vi "Pre Launch Init.vi"(11 "Keepalive Heartbeat in":refnum<class "Keepalive Heartbeat.lvclass">) -> (0 "error out":errorcluster, 3 "Keepalive Heartbeat out":refnum<class "Keepalive Heartbeat.lvclass">)   [LabVIEW 2021, in "WebSocket Actors.lvlib" / "Keepalive Heartbeat.lvclass"]
doc: "(<B>Filename</B>: Actor Framework.lvlib:Actor.lvclass:Pre Launch Init.vi)\n\nDefines behavior that occurs after the Launch Nested Actor method is invoked but before the actor's Actor Core method begins running.\n\nBy default, this method does nothing. A descendant class may override it to define behavior."
uses:
  Keepalive Heartbeat.lvclass
  Keepalive Heartbeat.lvclass/Keepalive Heartbeat.ctl
  <vilib>/ActorFramework/Actor/Actor.lvclass
  <userlib>/_OpenG.lib/error/error.llb/openg_error.lvlib
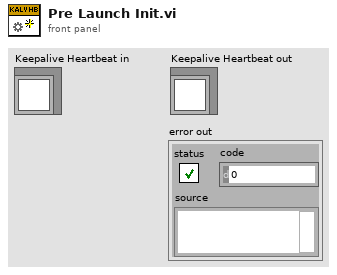
[diagram p1: front panel]
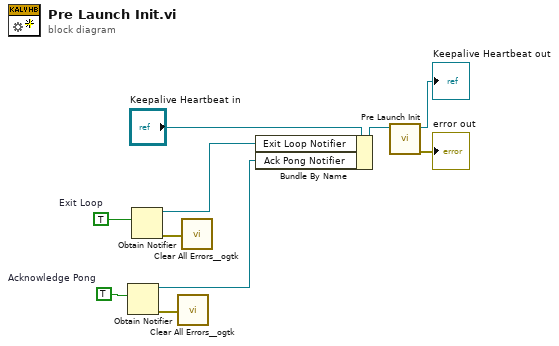
[diagram p0: block diagram]
diagram:
  w2 = TRUE  # Acknowledge Pong
  w7 = TRUE  # Exit Loop
  n1 = Obtain Notifier(notification data type=w2) -> (notifier out=w1:refnum<notifier>, error out=w3:errorcluster)  [unwired: 3 in, 1 out]
  n2 = Obtain Notifier(notification data type=w7) -> (notifier out=w5:refnum<notifier>, error out=w4:errorcluster)  [unwired: 3 in, 1 out]
  n3 = call <userlib>:"Clear All Errors__ogtk.vi"("Error In"=w3) -> ()  [unwired: 3 in, 1 out]
  n4 = call <userlib>:"Clear All Errors__ogtk.vi"("Error In"=w4) -> ()  [unwired: 3 in, 1 out]
  n5 = Bundle By Name(cluster="Keepalive Heartbeat in", "Exit Loop Notifier"=w5, "Ack Pong Notifier"=w1) -> (w6:refnum<class "Keepalive Heartbeat.lvclass">)
  n6 = call-parent "Pre Launch Init.vi"("Actor in"=w6) -> ("error out"=→"error out":errorcluster, "Actor out"=→"Keepalive Heartbeat out":refnum<class "Keepalive Heartbeat.lvclass">)  [unwired: 9 in]
